vi "Sign Data Example.vi"() -> ()   [LabVIEW 2016]
panel:
  out "signing time (ms)":dbl
  in  "Data to Sign":T1={"Data To Secure"={"Critical Data"={"Data to protect"="Important Data", "More data to protect"="More Important Data"}, "#attributes"={"signature"=""}}, "Some Other Data"={"Unprotected data"="Less Important Data"}}
  out "Validated Signed Data":T1
  out "Valid signature":bool
  out "Signed XML String":string
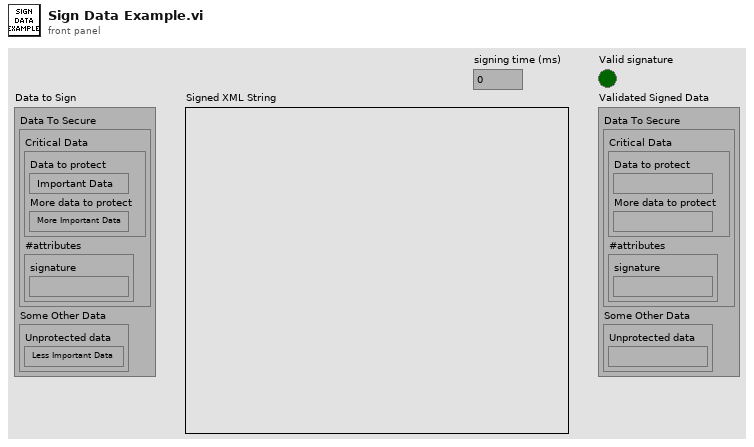
[diagram p1: front panel]
types:
  T1 = cluster{"Data To Secure":cluster{"Critical Data":cluster{"Data to protect":string, "More data to protect":string}, "#attributes":cluster{"signature":string}}, "Some Other Data":cluster{"Unprotected data":string}}
  T2 = cluster{"Data to protect":string, "More data to protect":string}
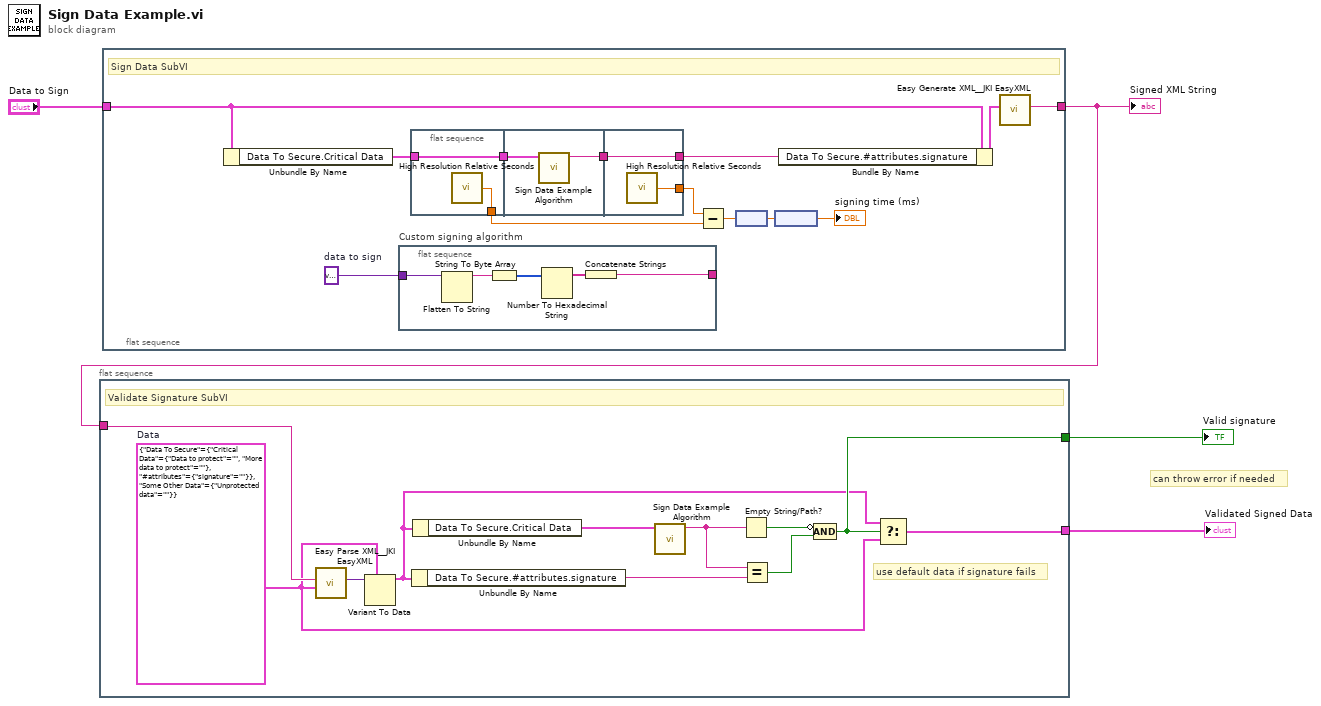
[diagram p0: block diagram]
diagram:
  # "can throw error if needed"
  n1 = flat-sequence {
    tunnel: w4 -> [w15]
    tunnel: [w9] -> w3
    tunnel: [w6] -> w2
    frame #0 {
      w7 = T1 {"Data To Secure"={"Critical Data"={"Data to protect"="", "More data to protect"=""}, "#attributes"={"signature"=""}}, "Some Other Data"={"Unprotected data"=""}}  # Data
      # "use default data if signature fails"
      # "Validate Signature SubVI"
      n2 = call <vilib>:"Easy Parse XML__JKI EasyXML.vi"("LabVIEW Data (Type)"=w7, "XML String"=w15) -> ("LabVIEW Data"=w14:variant)  [unwired: 8 in, 1 out]
      n3 = Variant To Data(type=w7, Variant=w14) -> (data=w8:T1)  [unwired: 1 in, 1 out]
      n4 = Unbundle By Name(w8) -> ("Data To Secure.#attributes.signature"=w5:string)
      n5 = Unbundle By Name(w8) -> ("Data To Secure.Critical Data"=w13:T2)
      n6 = call "Sign Data Example Algorithm.vi"("data"=w13) -> ("signature"=w12:string)  [unwired: 10 in]
      n7 = Empty String/Path?(string/path=w12) -> (empty?=w11:bool)
      n8 = Equal?(x=w12, y=w5) -> (x = y?=w10:bool)
      n9 = Compound Arithmetic op=AND(invert w11, w10) -> (w9:bool)
      n10 = Select(t=w8, s=w9, f=w7) -> (s? t:f=w6:T1)
    }
  }
  n11 = flat-sequence {
    tunnel: [w28] -> w4
    tunnel: "Data to Sign" -> [w27]
    frame #0 {
      w26 = variant  # data to sign
      # "Sign Data SubVI"
      n12 = Unbundle By Name(w27) -> ("Data To Secure.Critical Data"=w21:T2)
      n13 = flat-sequence "Custom signing algorithm" {
        tunnel: [w37] -> _
        tunnel: w26 -> [w35]
        frame #0 {
          n14 = Flatten To String(anything=w35) -> (data string=w36:string)  [unwired: 3 in, 2 out]
          n15 = String To Byte Array(string=w36) -> (unsigned byte array=w39:u8[])
          n16 = Number To Hexadecimal String(2:w39) -> (0:w38:string[])  [unwired: 1 in]
          n17 = Concatenate Strings(w38) -> (w37:string)
        }
      }
      n18 = flat-sequence {
        tunnel: w21 -> [w30]
        tunnel: [w30] -> w25
        tunnel: [w29] -> w19
        tunnel: [w32] -> w24
        tunnel: w25 -> [w31]
        tunnel: [w34] -> w22
        tunnel: w24 -> [w34]
        tunnel: [w33] -> w20
        frame #0 {
          n19 = call <vilib>:"High Resolution Relative Seconds.vi"() -> ("relative seconds"=w29:dbl)
        }
        frame #1 {
          n20 = call "Sign Data Example Algorithm.vi"("data"=w31) -> ("signature"=w32:string)  [unwired: 10 in]
        }
        frame #2 {
          n21 = call <vilib>:"High Resolution Relative Seconds.vi"() -> ("relative seconds"=w33:dbl)
        }
      }
      n22 = Subtract(x=w20, y=w19) -> (x-y=w18:dbl)
      n23 = node(w18) -> (w17:dbl[unit])
      n24 = node(w17) -> (→"signing time (ms)":dbl)
      n25 = Bundle By Name(cluster=w27, "Data To Secure.#attributes.signature"=w22) -> (w23:T1)
      n26 = call <vilib>:"Easy Generate XML__JKI EasyXML.vi"("LabVIEW Data"=w23) -> ("XML String"=w28:string)  [unwired: 9 in, 1 out]
    }
  }
  "Signed XML String" <- w4
  "Valid signature" <- w3
  "Validated Signed Data" <- w2
